vi "Display.vi"(8 "error in (no error)":errorcluster, 10 "ImageIndex":i32, 11 "Actor in":refnum<class "Actor.lvclass">) -> (0 "error out":errorcluster, 3 "Actor out":refnum<class "Actor.lvclass">)   [LabVIEW 2015, in "Actor.lvclass"]
uses:
  Actor.lvclass
  Actor.lvclass/Actor.ctl
  ImageOperaion/ImageOperation.lvclass
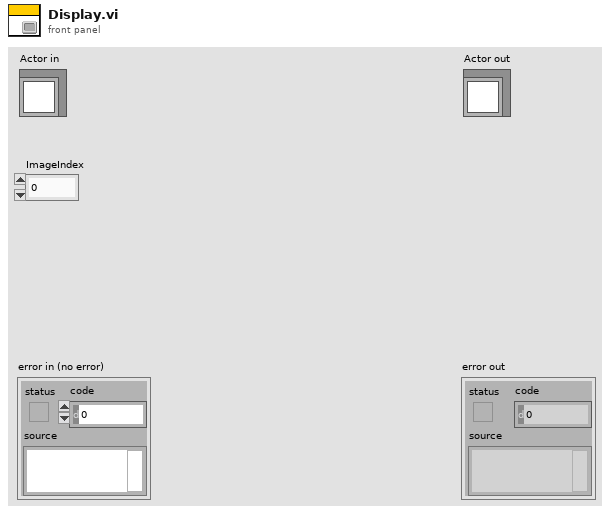
[diagram p1: front panel]
types:
  T1 = typedef "IMAQ Image.ctl" = refnum<image>
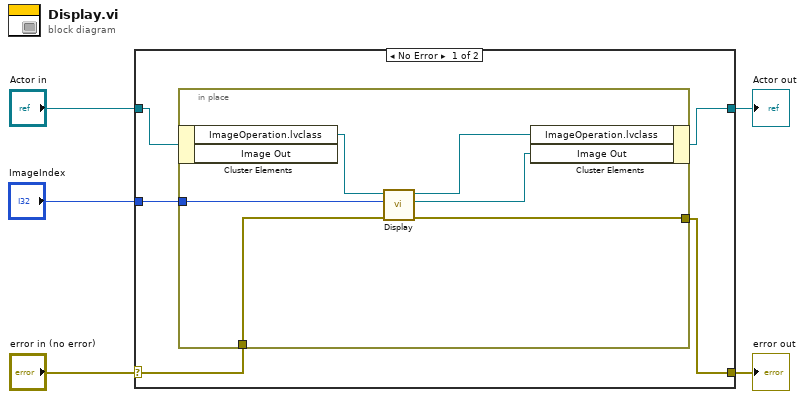
[diagram p0: block diagram]
diagram:
  n1 = case shown="No Error" "error in (no error)" {
    selector: "error in (no error)" -> [w8 w18]
    tunnel: [w7 w18] -> w4
    tunnel: [w6 w17] -> w2
    tunnel: "Actor in" -> [w10 w17]
    tunnel: "ImageIndex" -> [w9 _]
    frame No Error {
      n2 = in-place {
        in-place-border: w9 -> [w15]
        in-place-border: w8 -> [w13]
        in-place-border: [w12] -> w7
        n3 = in-place-cluster #1(w10) -> ("ImageOperation.lvclass"=w16:refnum<class "ImageOperation.lvclass">)  [unwired: 1 out]
        n4 = call "Display.vi"("error in (no error)"=w13, "ImageIndex"=w15, "ImageOperation in"=w16) -> ("error out"=w12:errorcluster, "Image Out"=w11:T1, "ImageOperation out"=w14:refnum<class "ImageOperation.lvclass">)  [unwired: 6 in]
        n5 = in-place-cluster #1("ImageOperation.lvclass"=w14, "Image Out"=w11) -> (w6:refnum<class "Actor.lvclass">)
      }
    }
    frame Error {
    }
  }
  "error out" <- w4
  "Actor out" <- w2
